vi "Actor Core.vi"(8 "error in":errorcluster, 11 "Nested in":refnum<class "gui.lvclass">) -> (0 "error out":errorcluster, 3 "Actor out":refnum<class "Actor.lvclass">)   [LabVIEW 2020, in "gui.lvlib" / "gui.lvclass"]
doc: "(<B>Filename</B>: Actor Framework.lvlib:Actor.lvclass:Actor Core.vi)\n\nReceives messages to the actor, reacts to them, and initiates any error handling that may shut the actor down.\n\nDescendant classes may override this VI to append parallel tasks for the actor to complete while it handles messages. Overrides use the Call Parent Method node."
uses:
  gui.lvclass
  C:/Program Files (x86)/National Instruments/LabVIEW 2020/vi.lib/ActorFramework/Actor/Actor.lvclass
  <vilib>/ActorFramework/Actor/Actor.lvclass
  <vilib>/ActorFramework/Actor/Actor.lvclass/Actor.ctl
  <vilib>/ActorFramework/Message Enqueuer/Message Enqueuer.lvclass/Message Enqueuer.ctl
  gui.lvclass/gui.ctl
  <vilib>/ActorFramework/Message Enqueuer/Init from Existing Queue.vi
  <vilib>/ActorFramework/Message Enqueuer/Enqueue.vi
  <vilib>/ActorFramework/Stop Msg/Stop Msg.lvclass
  C:/Program Files (x86)/National Instruments/LabVIEW 2020/vi.lib/ActorFramework/Message/Message.lvclass
  <vilib>/ActorFramework/Message Priority Queue/Priority Enqueue.vi
  <vilib>/ActorFramework/Message Enqueuer/Message Enqueuer.lvclass
panel:
  in  "Calibration":bool caption="Калибровка"
  in  "Connection":bool caption="Подключение"
  in  "Settings":bool caption="Настройки"
  in  "ViewData":bool caption="Показания"
  out "Tab Control":T1(tab)
  in  "Tab Control 2":enum32{"График", "Таблица"}(tab)
  out "Waveform Chart - Light":T2(graph)
  out "Table":string[][](table)
  in  "Close Button":bool
  in  "OK Button":bool
  in  "Find Sensor?":bool caption="Автопоиск"
  in  "Address":dbl caption="Modbus-адрес"
  in  "Parity enable?":bool caption="Контроль четности"
  in  "Baud":string(combo) caption="Скорость обмена, бод/с"
  in  "VISA":refnum<visa-resource-name> caption="COM-порт"
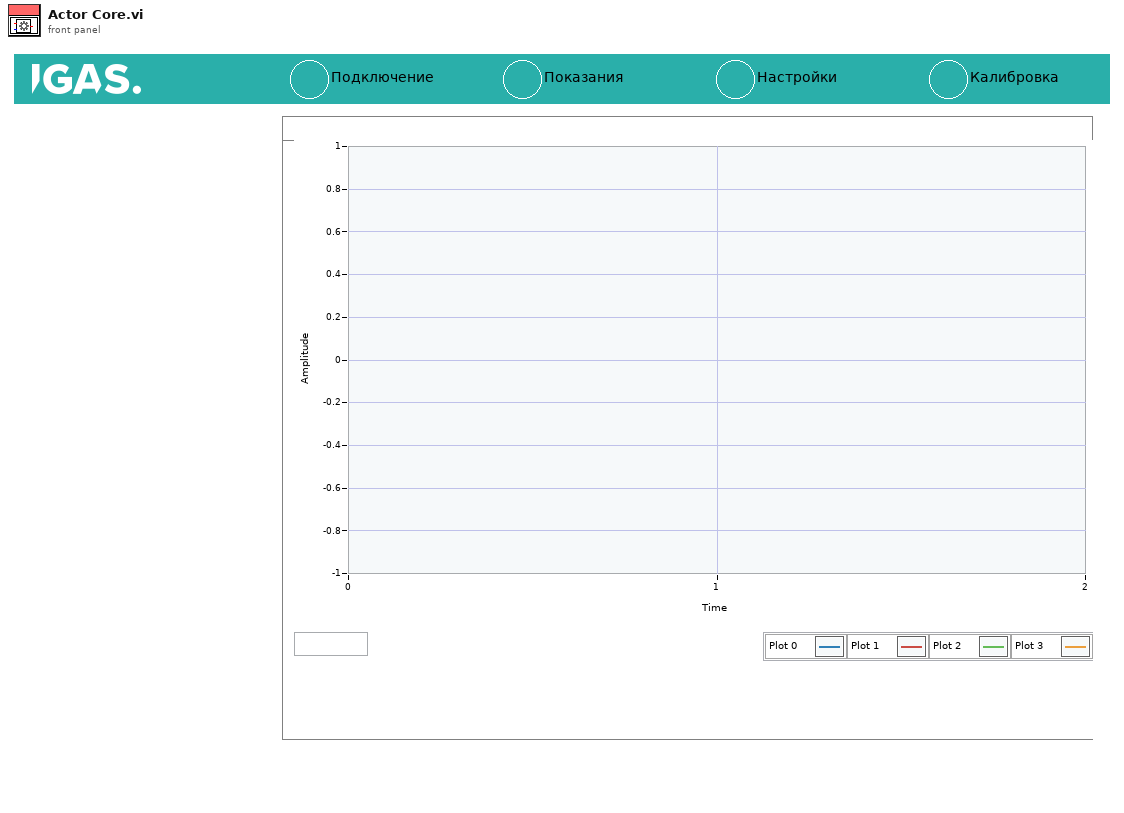
[diagram p1: front panel]
types:
  T1 = enum32{"Data", "Calibration", "Settings", "Connection"}
  T2 = cluster{"number":dbl, "number":dbl, "number":dbl, "number":dbl}
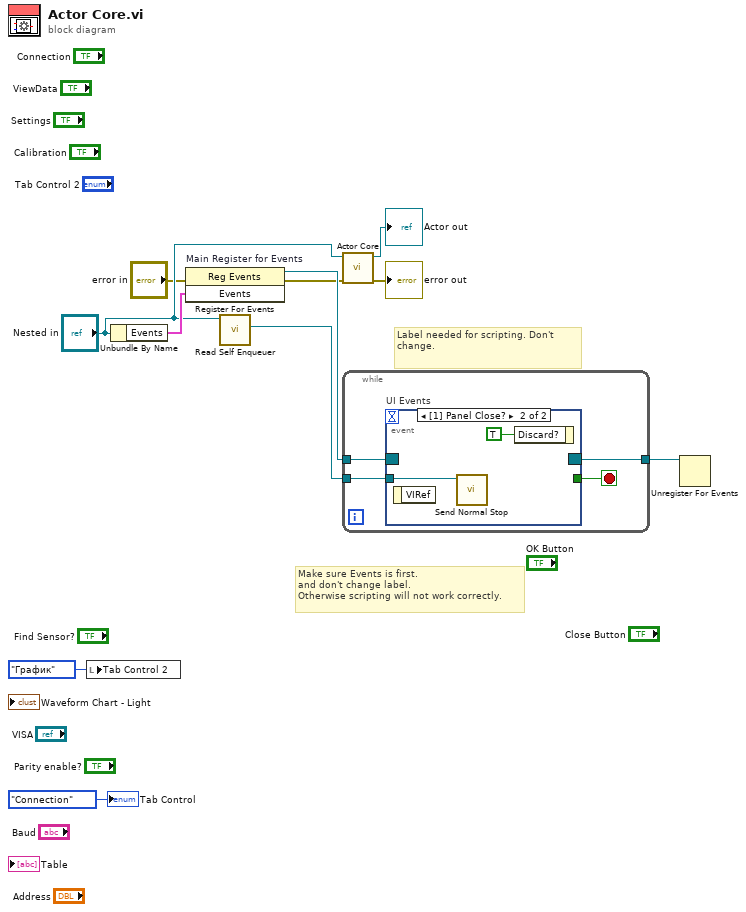
[diagram p0: block diagram]
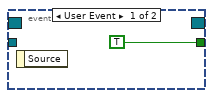
[diagram p2: hidden frame]
diagram:
  # "Label needed for scripting. Don't change."
  # "Make sure Events is first.\nand don't change label.\nOtherwise scripting will not work correctly."
  n1 = local write "Tab Control 2"(enum32{"График", "Таблица"}."График" ("Tab Control 2")) -> ()
  n2 = Unbundle By Name("Nested in") -> ("Events"=w8:cluster{"Stop":refnum<user-event>})
  n3 = register-events "Main Register for Events"(error in="error in", w8) -> (reference out=w9:refnum<event-registration>, error out=w3:errorcluster)  [unwired: 1 in]
  n4 = call <vilib>:"Read Self Enqueuer.vi"("Actor"="Nested in") -> ("Self Enqueuer"=w5:refnum<class "Message Enqueuer.lvclass">)  [unwired: 10 in]
  n5 = call-parent "Actor Core.vi"("error in"=w3, "Actor in"="Nested in") -> ("error out"=→"error out":errorcluster, "Actor out"=→"Actor out":refnum<class "Actor.lvclass">)  [unwired: 8 in]
  n6 = while {
    tunnel: w9 -> [w15]
    tunnel: [w13] -> w7
    tunnel: w5 -> [w12]
    stop <- w14 stop-if-true
    n7 = event "UI Events" shown="[1] Panel Close?" {
      selector: w15 -> [_ _]
      dyn-events: [_ _] -> w13
      timeout: _ -> [_ _]
      tunnel: [TRUE _] -> w14
      tunnel: w12 -> [_ w17]
      event User Event {
        n8 = event-data() -> ()  [unwired: 1 in, 1 out]
      }
      event Panel Close? {
        n9 = event-data() -> ()  [unwired: 1 in, 1 out]
        n10 = call <vilib>:"Send Normal Stop.vi"("Message Enqueuer"=w17) -> ()  [unwired: 10 in, 1 out]
        n11 = event-data("Discard?"=TRUE) -> ()  [unwired: 1 in, 1 out]
      }
    }
  }
  n12 = Unregister For Events(event registration refnum=w7) -> ()  [unwired: 1 in, 1 out]
  "Tab Control" <- T1."Connection" ("Tab Control")
